vi "CoerceBounds.vi"(0 "Zone in":refnum<class "Zone.lvclass">, 5 "centerPosition":dbl[](array[numeric]), 7 "lenght":dbl, 9 "width":dbl, 11 "error in (no error)":errorcluster) -> (4 "Zone out":refnum<class "Zone.lvclass">, 6 "lenghtBounds":dbl[](array[numeric]), 8 "widthBounds":dbl[](array[numeric]), 15 "error out":errorcluster)   [LabVIEW 2023, in "Zone.lvclass"]
uses:
  Zone.lvclass
  Zone.lvclass/Zone.ctl
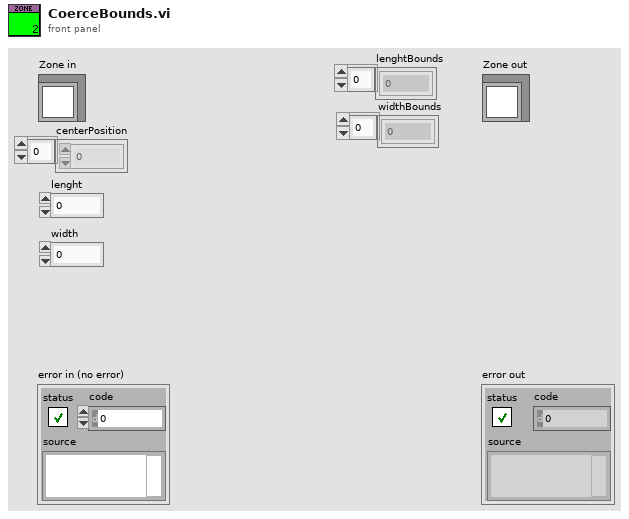
[diagram p1: front panel]
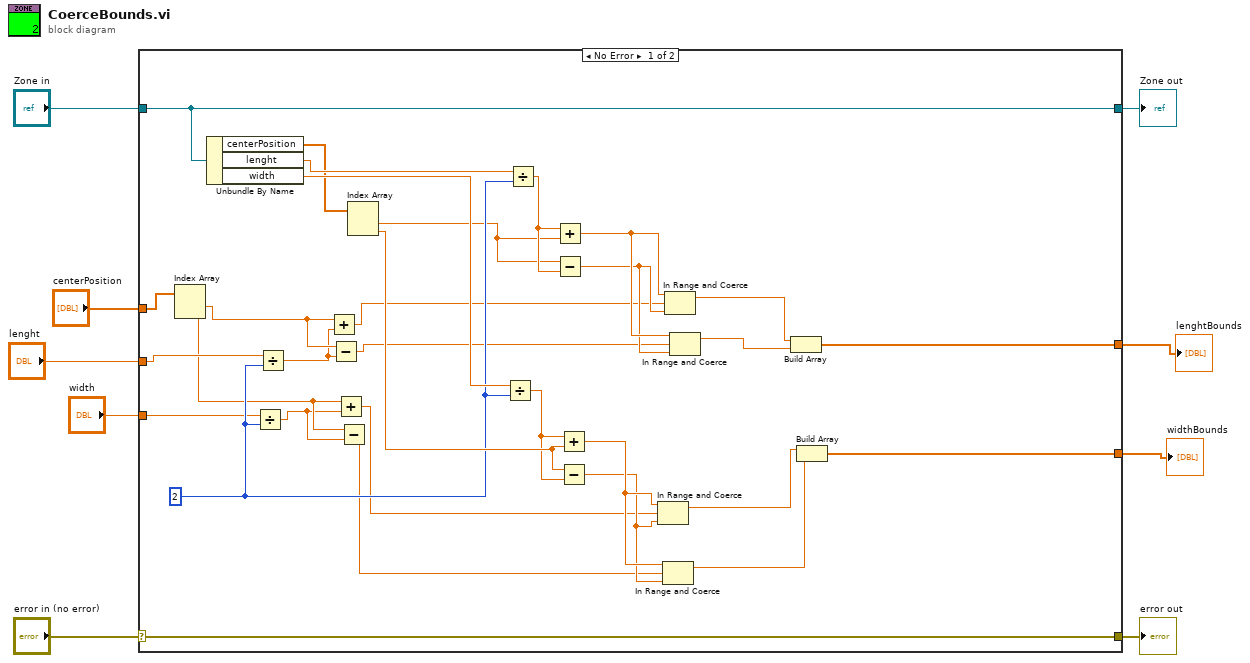
[diagram p0: block diagram]
diagram:
  n1 = case shown="No Error" "error in (no error)" {
    selector: "error in (no error)" -> [w40 w42]
    tunnel: [w40 w42] -> w8
    tunnel: [w39 w41] -> w6
    tunnel: "Zone in" -> [w39 w41]
    tunnel: "centerPosition" -> [w32 _]
    tunnel: "lenght" -> [w27 _]
    tunnel: "width" -> [w26 _]
    tunnel: [w13 _] -> w2
    tunnel: [w12 _] -> w1
    frame No Error {
      w33 = 2 ("y")
      n2 = Index Array(array=w32) -> (element #1=w25:dbl, element #2=w23:dbl)  [unwired: 2 in]
      n3 = Unbundle By Name(w39) -> ("centerPosition"=w36:dbl[], "lenght"=w38:dbl, "width"=w37:dbl)
      n4 = Divide(x=w26, y=w33) -> (x/y=w22:dbl)
      n5 = Divide(x=w27, y=w33) -> (x/y=w24:dbl)
      n6 = Add(x=w25, y=w24) -> (x+y=w21:dbl)
      n7 = Subtract(x=w25, y=w24) -> (x-y=w20:dbl)
      n8 = Add(x=w23, y=w22) -> (x+y=w19:dbl)
      n9 = Subtract(x=w23, y=w22) -> (x-y=w18:dbl)
      n10 = Index Array(array=w36) -> (element #1=w10:dbl, element #2=w35:dbl)  [unwired: 2 in]
      n11 = Divide(x=w37, y=w33) -> (x/y=w34:dbl)
      n12 = Divide(x=w38, y=w33) -> (x/y=w11:dbl)
      n13 = Add(x=w11, y=w10) -> (x+y=w31:dbl)
      n14 = Subtract(x=w10, y=w11) -> (x-y=w30:dbl)
      n15 = Add(x=w34, y=w35) -> (x+y=w29:dbl)
      n16 = Subtract(x=w35, y=w34) -> (x-y=w28:dbl)
      n17 = In Range and Coerce(upper limit=w29, x=w19, lower limit=w28) -> (coerced(x)=w15:dbl)  [unwired: 1 out]
      n18 = In Range and Coerce(upper limit=w29, x=w18, lower limit=w28) -> (coerced(x)=w14:dbl)  [unwired: 1 out]
      n19 = In Range and Coerce(upper limit=w31, x=w21, lower limit=w30) -> (coerced(x)=w17:dbl)  [unwired: 1 out]
      n20 = In Range and Coerce(upper limit=w31, x=w20, lower limit=w30) -> (coerced(x)=w16:dbl)  [unwired: 1 out]
      n21 = Build Array(w17, w16) -> (w13:dbl[])
      n22 = Build Array(w15, w14) -> (w12:dbl[])
    }
    frame Error {
    }
  }
  "error out" <- w8
  "Zone out" <- w6
  "widthBounds" <- w1
  "lenghtBounds" <- w2
